vi "CT-Constrain Random Phase.vi"(0 "HCT Runtime":T1, 5 "Fs (Hz)":dbl, 7 "Max peak factor":dbl, 9 "Max mod depth":dbl) -> (4 "Phase":dbl[](array[numeric]), 15 "error out":errorcluster)   [LabVIEW 2015]
uses:
  CT-Runtime Data.ctl
  Utility VIs/Math VIs/LinSpace (x0-dx-npts).vi
  <vilib>/Analysis/2dsp.llb/Real FFT.vi
  <vilib>/Analysis/5stat.llb/RMS (DBL).vi
  <vilib>/Analysis/NI_AALBase.lvlib
  <vilib>/Analysis/NI_AALPro.lvlib
panel:
  out "tries":i32
  out "mod depth":dbl
  out "peak factor":dbl
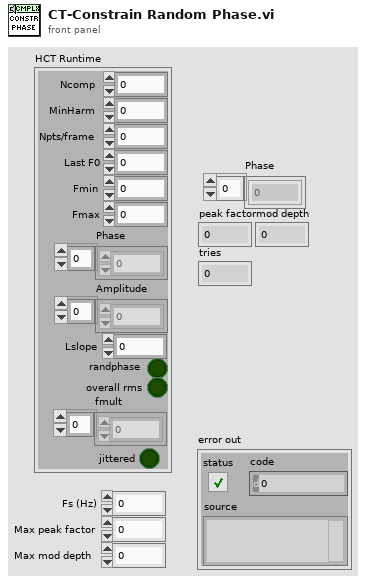
[diagram p1: front panel]
types:
  T1 = typedef "CT-Runtime Data.ctl" = cluster{"Ncomp":i32, "MinHarm":i32, "Phase":dbl[], "Amplitude":dbl[], "Npts/frame":i32, "Last F0":dbl, "Fmin":dbl, "Fmax":dbl, "Lslope":dbl, "randphase":bool, "overall rms":bool, "fmult":dbl[], "jittered":bool}
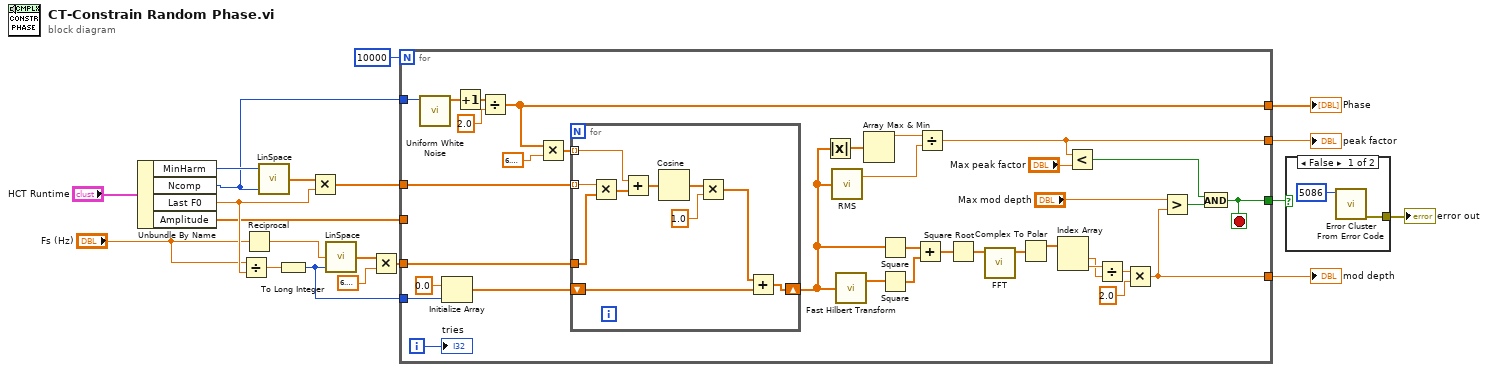
[diagram p0: block diagram]
diagram:
  n1 = Unbundle By Name("HCT Runtime") -> ("MinHarm"=w19:i32, "Ncomp"=w8:i32, "Last F0"=w16:dbl, "Amplitude"=w12:dbl[])
  n2 = Divide(x="Fs (Hz)", y=w16) -> (x/y=w18:dbl)
  n3 = Reciprocal(x="Fs (Hz)") -> (1/x=w14:dbl)
  n4 = call-poly "LinSpace.vi"("npts"=w8, "x0"=w19) -> ("Array"=w17:dbl[])  [unwired: 2 in, 1 out]
  n5 = To Long Integer(number=w18) -> (32bit integer=w7:i32)
  n6 = Multiply(x=w17, y=w16) -> (x*y=w13:dbl[])
  n7 = call-poly "LinSpace.vi"("npts"=w7, "dx"=w14) -> ("Array"=w11:dbl[])  [unwired: 2 in, 1 out]
  n8 = Multiply(x=w11, y=6.283185307179586) -> (x*y=w9:dbl[])
  n9 = for {
    N: 10000 -> [_]
    tunnel: w13 -> [w55]
    tunnel: w12 -> [_]
    tunnel: w9 -> [w54]
    tunnel: w8 -> [w53]
    tunnel: w7 -> [w52]
    tunnel: [w25] -> w6
    tunnel: [w34] -> w4
    tunnel: [w31] -> w3
    tunnel: [w28] -> w2
    i -> [w21]
    stop <- w28 stop-if-true
    n10 = call <vilib>:"Uniform White Noise.vi"("samples"=w53) -> ("uniform white noise"=w27:dbl[])  [unwired: 9 in, 1 out]
    n11 = Initialize Array(0.0 ("element"), w52) -> (w50:dbl[])
    n12 = Increment(x=w27) -> (x+1=w26:dbl[])
    n13 = Divide(x=w26, y=2.0) -> (x/y=w25:dbl[])
    n14 = Multiply(x=w25, y=6.283185307179586) -> (x*y=w23:dbl[])
    n15 = for {
      tunnel: w55 -> [w65] mode=indexing
      tunnel: w54 -> [w64]
      tunnel: w23 -> [w61] mode=indexing
      shift-right: [w57] -> w46
      shift-left: w50 -> [w58]
      n16 = Multiply(x=w65, y=w64) -> (x*y=w62:dbl[])
      n17 = Add(x=w61, y=w62) -> (x+y=w63:dbl[])
      n18 = Cosine(x=w63) -> (cos(x)=w60:dbl[])
      n19 = Multiply(x=w60, y=1.0) -> (x*y=w59:dbl[])
      n20 = Add(x=w59, y=w58) -> (x+y=w57:dbl[])
    }
    n21 = Absolute Value(x=w46) -> (abs(x)=w49:dbl[])
    n22 = call-poly <vilib>:"RMS.vi"("X"=w46) -> ("rms value"=w47:dbl)  [unwired: 1 out]
    n23 = call <vilib>:"Fast Hilbert Transform.vi"("X"=w46) -> ("Hilbert{X}"=w45:dbl[])  [unwired: 1 out]
    n24 = Array Max & Min(array=w49) -> (max value=w48:dbl)  [unwired: 3 out]
    n25 = Square(x=w46) -> (x^2=w44:dbl[])
    n26 = Square(x=w45) -> (x^2=w43:dbl[])
    n27 = Add(x=w44, y=w43) -> (x+y=w42:dbl[])
    n28 = Divide(x=w48, y=w47) -> (x/y=w34:dbl)
    n29 = Square Root(x=w42) -> (sqrt(x)=w41:dbl[])
    n30 = call-poly <vilib>:"FFT.vi"("X"=w41) -> ("FFT {X}"=w40:cdb[])  [unwired: 9 in, 1 out]
    n31 = Complex To Polar(r * e^(i*theta)=w40) -> (r=w36:dbl[])  [unwired: 1 out]
    n32 = Index Array(array=w36) -> (element #1=w38:dbl, element #2=w39:dbl)  [unwired: 2 in]
    n33 = Less?(x=w34, y="Max peak factor") -> (x < y?=w29:bool)
    n34 = Divide(x=w39, y=w38) -> (x/y=w37:dbl)
    n35 = Multiply(x=w37, y=2.0) -> (x*y=w31:dbl)
    n36 = Greater?(x="Max mod depth", y=w31) -> (0:w30:bool)
    n37 = And(x=w29, y=w30) -> (x .and. y?=w28:bool)
    "tries" <- w21
  }
  "Phase" <- w6
  "peak factor" <- w4
  "mod depth" <- w3
  n38 = case shown="False" w2 {
    tunnel: [w67 _] -> w1
    frame False {
      n39 = call <vilib>:"Error Cluster From Error Code.vi"("error code (0)"=5086) -> ("error out"=w67:errorcluster)  [unwired: 8 in]
    }
    frame True {
    }
  }
  "error out" <- w1
